vi "Nachkommastellen begrenzen.vi"(9 "Nachkommastellen":i16, 11 "DBL-String mit Deziamlpunkt":string) -> (3 "Anzeigestring mit Komma":string)   [LabVIEW 2020, in "Anlagenuebersicht.lvlib" / "VisBx Anzeige.lvlib"]
uses:
  VisBx Anzeige.lvlib
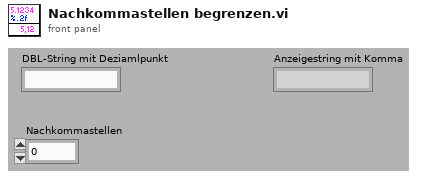
[diagram p1: front panel]
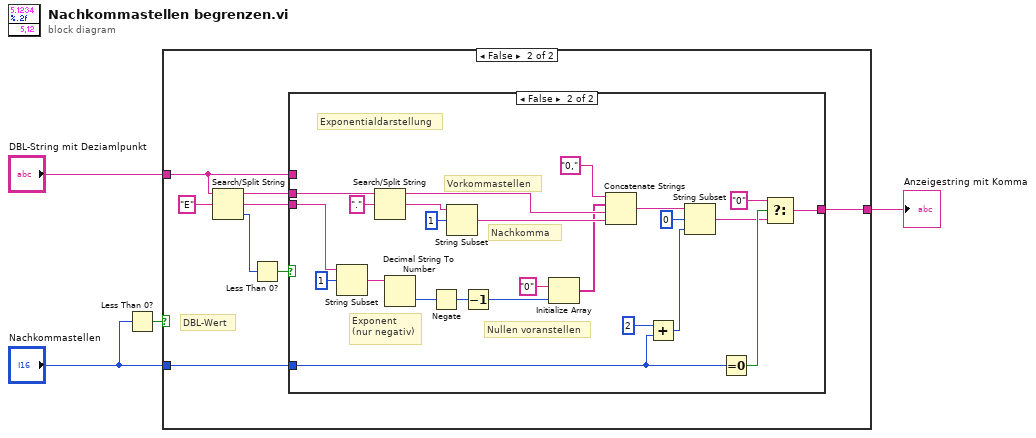
[diagram p0: block diagram]
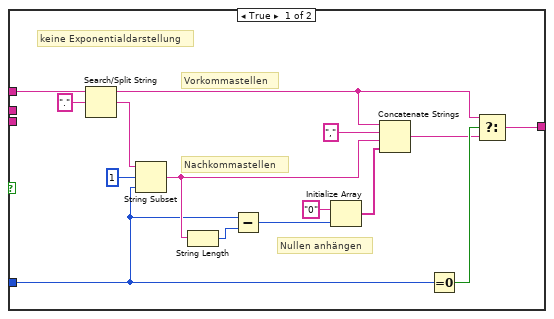
[diagram p3: hidden frame]
diagram:
  n1 = Less Than 0?(x="Nachkommastellen") -> (x < 0?=w1:bool)
  n2 = case shown="False" w1 {
    tunnel: [w5 w13] -> w4
    tunnel: "Nachkommastellen" -> [_ w12]
    tunnel: "DBL-String mit Deziamlpunkt" -> [w5 w9]
    frame True {
      # "kein DBL-Wert"
    }
    frame False {
      # "DBL-Wert"
      n3 = Search/Split String(string=w9, search string/char (-)="E" ("Nach String/Zeichen suchen (-)")) -> (substring before match=w7:string, match + rest of string=w6:string, offset of match=w11:i32)  [unwired: 1 out]
      n4 = Less Than 0?(x=w11) -> (x < 0?=w8:bool)
      n5 = case shown="False" w8 {
        tunnel: [w15 w47] -> w13
        tunnel: w12 -> [w19 w34]
        tunnel: w9 -> [w20 _]
        tunnel: w7 -> [_ w35]
        tunnel: w6 -> [_ w45]
        frame True {
          # "Vorkommastellen"
          # "Nachkommastellen"
          # "keine Exponentialdarstellung"
          # "Nullen anhängen"
          n6 = Search/Split String(string=w20, search string/char (-)="." ("Regulärer Ausdruck")) -> (substring before match=w17:string, match + rest of string=w28:string)  [unwired: 2 out]
          n7 = String Subset(string=w28, offset (0)=1 ("Offset (0)"), length (rest)=w19) -> (substring=w25:string)
          n8 = String Length(string=w25) -> (length=w24:i32)
          n9 = Subtract(x=w19, y=w24) -> (x-y=w23:i32)
          n10 = Initialize Array("0", w23) -> (w21:string[])
          n11 = Concatenate Strings(w17, "," ("String"), w25, w21) -> (w16:string)
          n12 = Equal To 0?(x=w19) -> (x = 0?=w18:bool)
          n13 = Select(t=w17, s=w18, f=w16) -> (s? t:f=w15:string)
        }
        frame False {
          # "Nachkomma"
          # "Vorkommastellen"
          # "Exponent\n(nur negativ)"
          # "Exponentialdarstellung"
          # "Nullen voranstellen"
          n14 = String Subset(string=w45, offset (0)=1 ("Offset (0)")) -> (substring=w43:string)  [unwired: 1 in]
          n15 = Search/Split String(string=w35, search string/char (-)="." ("Regulärer Ausdruck")) -> (substring before match=w48:string, match + rest of string=w52:string)  [unwired: 2 out]
          n16 = Decimal String To Number(string=w43) -> (number=w38:i32)  [unwired: 2 in, 1 out]
          n17 = Negate(x=w38) -> (-x=w37:i32)
          n18 = String Subset(string=w52, offset (0)=1 ("Offset (0)")) -> (substring=w42:string)  [unwired: 1 in]
          n19 = Decrement(x=w37) -> (x-1=w36:i32)
          n20 = Initialize Array("0", w36) -> (w41:string[])
          n21 = Concatenate Strings("0,", w41, w48, w42) -> (w30:string)
          n22 = Add(x=i16 2, y=w34) -> (x+y=w32:i16)
          n23 = String Subset(string=w30, offset (0)=0 ("Offset (0)"), length (rest)=w32) -> (substring=w29:string)
          n24 = Equal To 0?(x=w34) -> (x = 0?=w49:bool)
          n25 = Select(t="0", s=w49, f=w29) -> (s? t:f=w47:string)
        }
      }
    }
  }
  "Anzeigestring mit Komma" <- w4
